vi "Feature Name.vi"() -> (2 "Feature name":string, 3 "Out":bool)   [LabVIEW 2015]
uses:
  Control Button/Exit.ctl
  Control PB/Next_.ctl
panel:
  in  "Feature list":string(combo)="Ionizer"
  in  "Next":T1
  in  "Exit":T2
  # "Add Feature List"
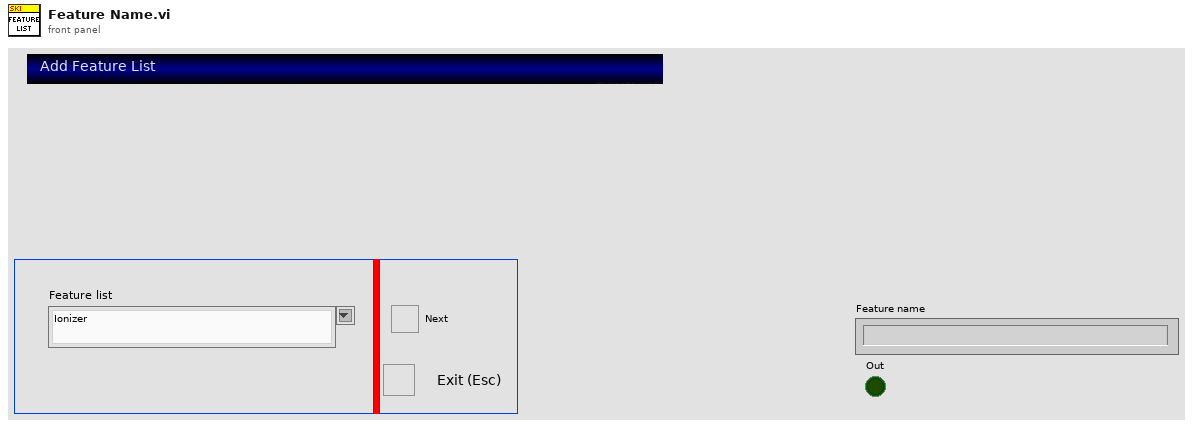
[diagram p1: front panel]
types:
  T1 = typedef "Next_.ctl" = bool
  T2 = typedef "Exit.ctl" = bool
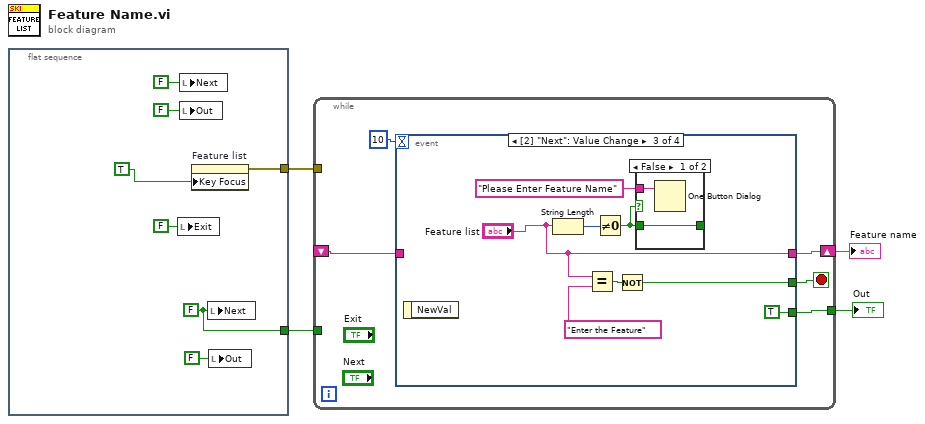
[diagram p0: block diagram]
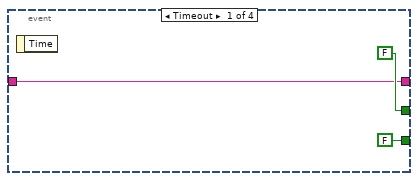
[diagram p2: hidden frame]
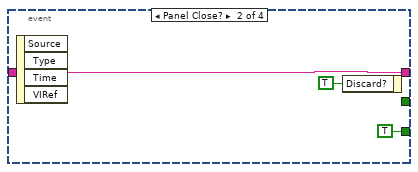
[diagram p3: hidden frame]
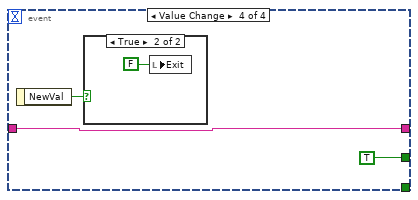
[diagram p5: hidden frame]
diagram:
  n1 = flat-sequence {
    tunnel: [w8] -> w2
    tunnel: [w5] -> w1
    frame #0 {
      w8 = T1 FALSE ("Next")
      n2 = local write "Exit"(FALSE ("Exit")) -> ()
      n3 = local write "Next"(T1 FALSE ("Next")) -> ()
      n4 = local write "Out"(FALSE ("Out")) -> ()
      n5 = property on="Feature list" class="CmbBox"("Key Focus"=TRUE) -> (error out=w5:errorcluster)  [unwired: 2 in, 1 out]
      n6 = local write "Next"(w8) -> ()
      n7 = local write "Out"(FALSE ("Out")) -> ()
    }
  }
  n8 = while {
    tunnel: [w14] -> w3
    tunnel: w2 -> [_]
    shift-right: [w15] -> w4
    shift-left: _ -> [w12]
    tunnel: w1 -> [_]
    stop <- w16 stop-if-true
    n9 = event shown="[2] \"Next\": Value Change" {
      selector: _ -> [_ _ _ _]
      dyn-events: _ -> [_ _ _ _]
      timeout: 10 -> [_ _ _ _]
      tunnel: [FALSE _ w25 TRUE] -> w16
      tunnel: [w17 w20 "Feature list" w34] -> w15
      tunnel: [T1 FALSE ("NewVal") T1 TRUE ("NewVal") T1 TRUE ("NewVal") _] -> w14
      tunnel: w12 -> [w17 w20 _ w34]
      event Timeout {
        n10 = event-data() -> ()  [unwired: 1 in, 1 out]
      }
      event Panel Close? {
        n11 = event-data() -> ()  [unwired: 1 in, 4 out]
        n12 = event-data("Discard?"=TRUE) -> ()  [unwired: 1 in, 1 out]
      }
      event Value Change {
        n13 = event-data() -> ()  [unwired: 1 in, 1 out]
        n14 = String Length(string="Feature list") -> (length=w30:i32)
        n15 = Equal?(x="Feature list", y="Enter the Feature") -> (x = y?=w26:bool)
        n16 = Not Equal To 0?(x=w30) -> (x != 0?=w28:bool)
        n17 = Not(x=w26) -> (.not. x?=w25:bool)
        n18 = case shown="False" w28 {
          tunnel: "Please Enter Feature Name" ("message") -> [w32 _]
          tunnel: [w31 w33] -> _
          tunnel: w28 -> [w31 w33]
          frame False {
            n19 = One Button Dialog(message=w32) -> ()  [unwired: 1 in, 1 out]
          }
          frame True {
          }
        }
      }
      event Value Change {
        n20 = event-data() -> ("NewVal"=w35:T2)  [unwired: 1 in]
        n21 = case shown="True" w35 {
          frame False {
          }
          frame True {
            n22 = local write "Exit"(T1 FALSE ("Next")) -> ()
          }
        }
      }
    }
  }
  "Feature name" <- w4
  "Out" <- w3
